vi "Highlight the Error GU Cell.vi"(7 "Top VI":refnum<vi>, 8 "error in":errorcluster, 9 "Error Cell":T2(array[cluster]), 11 "GU Arrange List":refnum<vi>) -> (0 "error out":errorcluster, 1 "Error Cell  Out":T2(array[cluster]))   [LabVIEW 2020, in "GUCalibration2.lvlib"]
uses:
  GUCalibration2.lvlib
  Controls/GU Arrange Check Rule.ctl
  25c2320b-937b-4a15-b365-74d593e864c5.vi
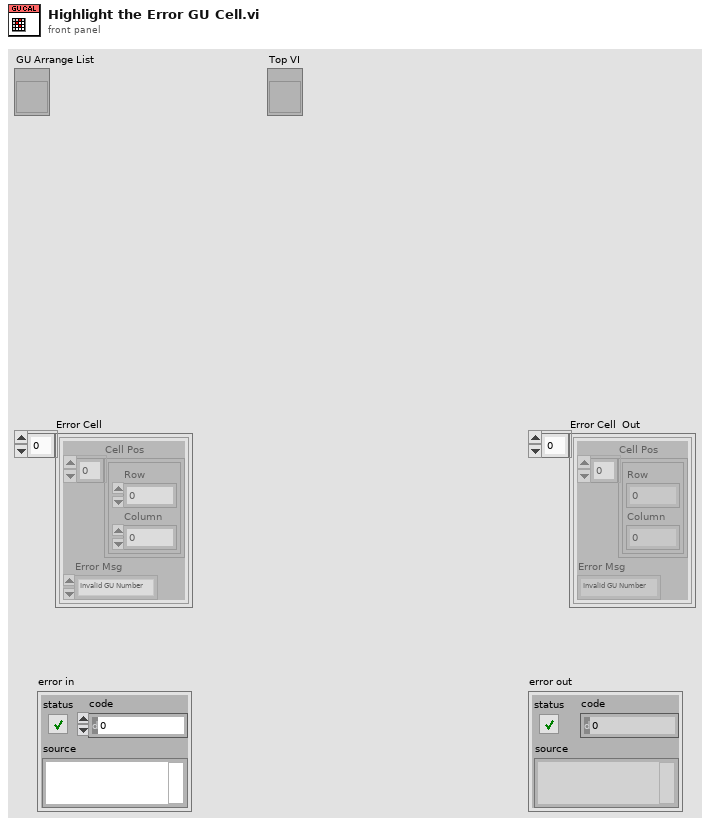
[diagram p1: front panel]
types:
  T1 = typedef "GUCalibration2.lvlib/GU Arrange Check Rule.ctl" = enum16{"Invalid GU Number", "GU Number Conflict"}
  T2 = cluster{"Cell Pos":cluster{"Row":i32, "Column":i32}[], "Error Msg":T1}[]
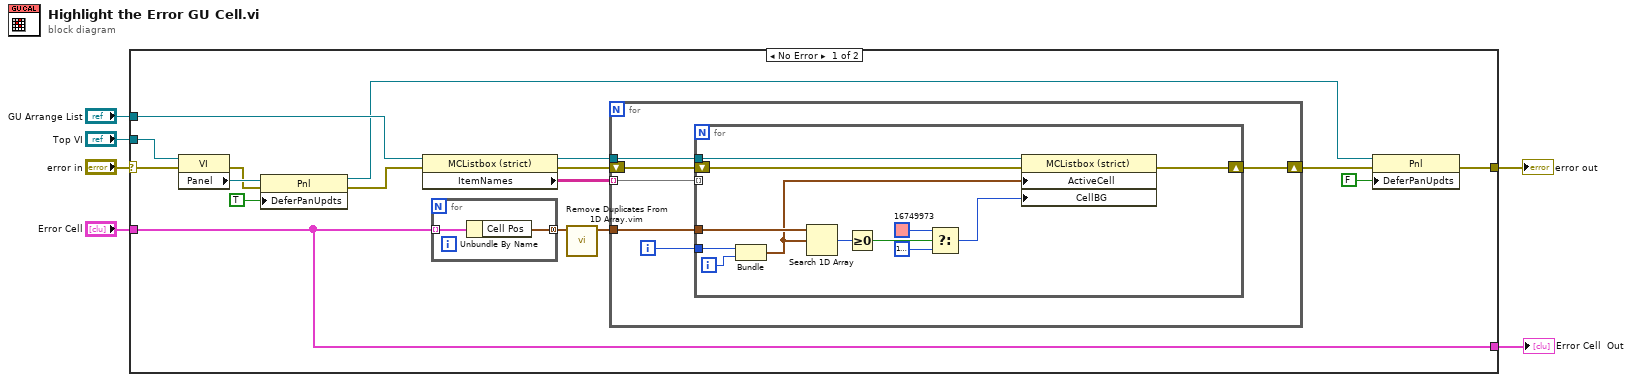
[diagram p0: block diagram]
diagram:
  n1 = case shown="No Error" "error in" {
    selector: "error in" -> [w15 w45]
    tunnel: "GU Arrange List" -> [w23 _]
    tunnel: [w10 w45] -> w5
    tunnel: "Error Cell" -> [w17 w44]
    tunnel: [w17 w44] -> w2
    tunnel: "Top VI" -> [w9 _]
    frame No Error {
      n2 = property class="VI"(reference=w9, error in=w15) -> (error out=w14:errorcluster, "Panel"=w16:refnum<vi>)  [unwired: 1 out]
      n3 = property class="Pnl"(reference=w16, error in=w14, "DeferPanUpdts"=TRUE ("Defer Panel Updates")) -> (reference out=w8:refnum<vi>, error out=w12:errorcluster)
      n4 = property class="MCListbox (strict)"(reference=w23, error in=w12) -> (reference out=w22:refnum<vi>, error out=w21:errorcluster, "ItemNames"=w20:string[][])
      n5 = for {
        tunnel: w17 -> [w25] mode=indexing
        tunnel: [w24] -> w19 mode=concatenating
        n6 = Unbundle By Name(w25) -> ("Cell Pos"=w24:cluster{"Row":i32, "Column":i32}[])
      }
      n7 = call "Remove Duplicates From 1D Array.vim"("array"=w19) -> ("array with duplicates removed"=w18:cluster{"Row":i32, "Column":i32}[])  [unwired: 10 in]
      n8 = for {
        tunnel: w22 -> [w31]
        tunnel: w20 -> [w29] mode=indexing
        tunnel: w18 -> [w28]
        shift-right: [w26] -> w11
        shift-left: w21 -> [w30]
        i -> [w27]
        n9 = for {
          tunnel: w31 -> [w43]
          tunnel: w29 -> [_] mode=indexing
          tunnel: w28 -> [w41]
          tunnel: w27 -> [w40]
          shift-right: [w32] -> w26
          shift-left: w30 -> [w42]
          i -> [w39]
          n10 = Bundle(w40, w39) -> (w33:cluster{i32, i32})  [unwired: 1 in]
          n11 = Search 1D Array(1D array=w41, element=w33) -> (index of element=w38:i32)  [unwired: 1 in]
          n12 = Greater Or Equal To 0?(x=w38) -> (x >= 0?=w37:bool)
          n13 = Select(t=u32 16749973, s=w37, f=u32 16777225) -> (s? t:f=w35:u32)
          n14 = property class="MCListbox (strict)"(reference=w43, error in=w42, "ActiveCell"=w33, "CellBG"=w35) -> (error out=w32:errorcluster)  [unwired: 1 out]
        }
      }
      n15 = property class="Pnl"(reference=w8, error in=w11, "DeferPanUpdts"=FALSE ("Defer Panel Updates")) -> (error out=w10:errorcluster)  [unwired: 1 out]
    }
    frame Error {
    }
  }
  "error out" <- w5
  "Error Cell  Out" <- w2
